vi "Temperature Warnings.vi"() -> ()   [LabVIEW 2012]
doc: "In this exercise, you convert the weather data cluster into a type definition."
uses:
  Weather Data.ctl
panel:
  out "Weather Data Out":T1={"Current Temperature"=0.0, "Max Temperature"=0.0, "Min Temperature"=0.0, "Temperature Warning?"=FALSE, "Temperature Warning Text"="No Warning", "Units"=0} {"Units" items=["Celsius", "Fahrenheit"]}
  in  "Weather Data In":T1={"Current Temperature"=0.0, "Max Temperature"=0.0, "Min Temperature"=0.0, "Temperature Warning?"=FALSE, "Temperature Warning Text"="No Warning", "Units"=0} {"Units" items=["Celsius", "Fahrenheit"]}
  out "Error Out":errorcluster
  in  "Error In":errorcluster
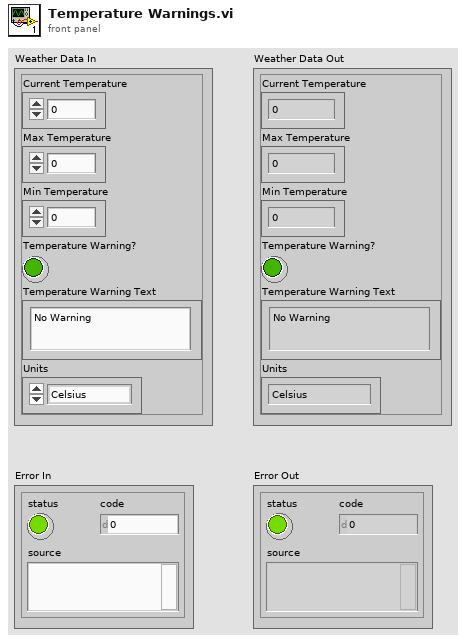
[diagram p1: front panel]
types:
  T1 = typedef "Weather Data.ctl" = cluster{"Current Temperature":dbl, "Max Temperature":dbl, "Min Temperature":dbl, "Temperature Warning?":bool, "Temperature Warning Text":string, "Units":u16}
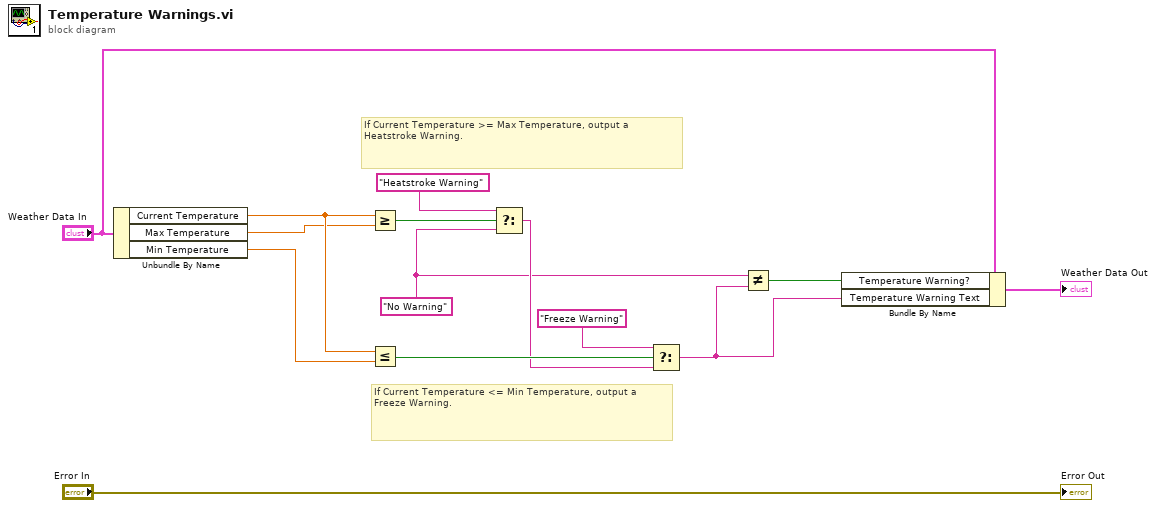
[diagram p0: block diagram]
diagram:
  w1 = "No Warning" ("f")
  # "If Current Temperature <= Min Temperature, output a Freeze Warning."
  # "If Current Temperature >= Max Temperature, output a Heatstroke Warning."
  n1 = Unbundle By Name("Weather Data In") -> ("Current Temperature"=w13:dbl, "Max Temperature"=w12:dbl, "Min Temperature"=w11:dbl)
  n2 = Greater Or Equal?(x=w13, y=w12) -> (x >= y?=w6:bool)
  n3 = Less Or Equal?(x=w13, y=w11) -> (x <= y?=w3:bool)
  n4 = Select(t="Heatstroke Warning", s=w6, f=w1) -> (s? t:f=w2:string)
  n5 = Select(t="Freeze Warning", s=w3, f=w2) -> (s? t:f=w10:string)
  n6 = Not Equal?(x=w1, y=w10) -> (x != y?=w9:bool)
  n7 = Bundle By Name(cluster="Weather Data In", "Temperature Warning?"=w9, "Temperature Warning Text"=w10) -> (→"Weather Data Out":T1)
  "Error Out" <- "Error In"
